vi "Configure Setpoint and Ramp.vi"(0 "VISA resource name":refnum<visa-resource-name>, 1 "Enable Setpoint Ramping  (F: Disable)":bool, 2 "Ramp Rate (0.0)":dbl format="%.3f", 5 "Output's Control Loop (1:1)":u16(ring)=1 items=["1"=1, "2"=2, "3"=3, "4"=4], 7 "Setpoint (0.00000)":dbl format="%.5f", 11 "error in (no error)":errorcluster) -> (4 "VISA resource name out":refnum<visa-resource-name>, 15 "error out":errorcluster)   [LabVIEW 2016, in "Lake Shore 350.lvlib"]
doc: "Configures the Setpoint and Setpoint Ramping function. The Setpoint parameter is used to set the desired load temperature for a control loop."
uses:
  Lake Shore 350.lvlib
  Instance           2 35Saved   Configure Setpoint and Ramp .vi
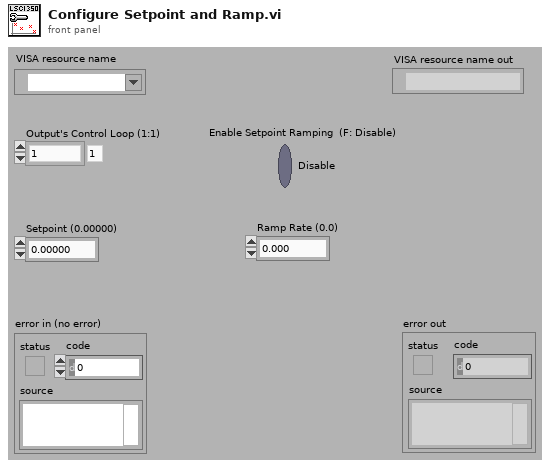
[diagram p1: front panel]
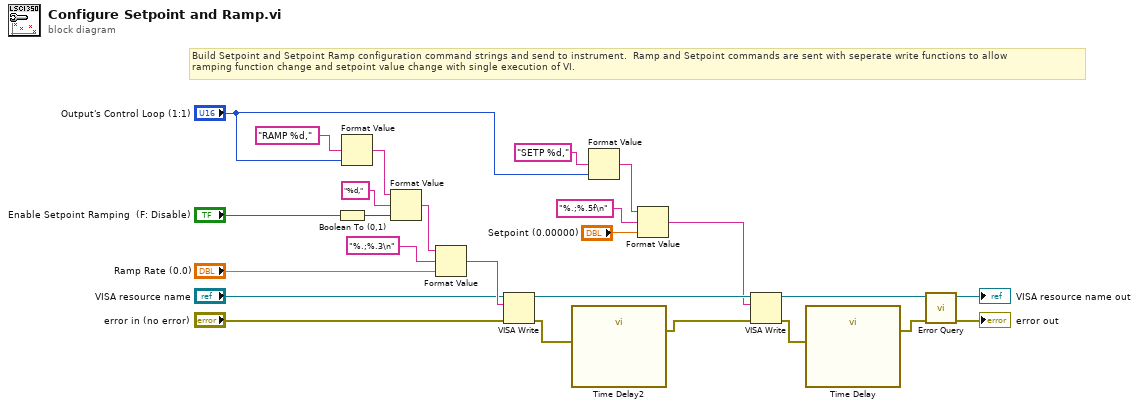
[diagram p0: block diagram]
diagram:
  # "Build Setpoint and Setpoint Ramp configuration command strings and send to instrument.  Ramp and Setpoint commands are sent with seperate write functions to allow\nramping function change and setpoint value change with single execution of VI."
  n1 = Boolean To (0,1)(Boolean="Enable Setpoint Ramping  (F: Disable)") -> (0, 1=w15:i16)
  n2 = Format Value(format string="RAMP %d,", value (0)="Output's Control Loop (1:1)") -> (output string=w9:string)  [unwired: 1 in]
  n3 = Format Value(string ("")=w9, format string="%d,", value (0)=w15) -> (output string=w13:string)
  n4 = Format Value(string ("")=w13, format string="%.;%.3\n", value (0)="Ramp Rate (0.0)") -> (output string=w7:string)
  n5 = VISA Write(VISA resource name="VISA resource name", write buffer=w7, error in (no error)="error in (no error)") -> (VISA resource name out=w6:refnum<visa-resource-name>, error out=w5:errorcluster)  [unwired: 1 out]
  n6 = call "Time Delay2"("error in (no error)"=w5) -> ("error out"=w4:errorcluster)  [unwired: 10 in]
  n7 = Format Value(format string="SETP %d,", value (0)="Output's Control Loop (1:1)") -> (output string=w17:string)  [unwired: 1 in]
  n8 = Format Value(string ("")=w17, format string="%.;%.5f\n", value (0)="Setpoint (0.00000)") -> (output string=w3:string)
  n9 = VISA Write(VISA resource name=w6, write buffer=w3, error in (no error)=w4) -> (VISA resource name out=w25:refnum<visa-resource-name>, error out=w22:errorcluster)  [unwired: 1 out]
  n10 = call "Time Delay"("error in (no error)"=w22) -> ("error out"=w21:errorcluster)  [unwired: 10 in]
  n11 = call "Error Query.vi"("error in (no error)"=w21, "VISA resource name"=w25) -> ("error out"=→"error out":errorcluster, "VISA resource name out"=→"VISA resource name out":refnum<visa-resource-name>)  [unwired: 7 in, 1 out]
